vi "ppanel_DO_get_current_count_rates.vi"(8 "error in (no error)":errorcluster, 11 "hydraharp_panel in":refnum<class "picoharp_panel.lvclass">) -> (0 "error out":errorcluster, 3 "hydraharp_panel out":refnum<class "picoharp_panel.lvclass">)   [LabVIEW 2015, in "picoharp_panel.lvclass"]
uses:
  picoharp_panel.lvclass
  picoharp/picoharp.lvclass
  UI/panel_class/panel.lvclass
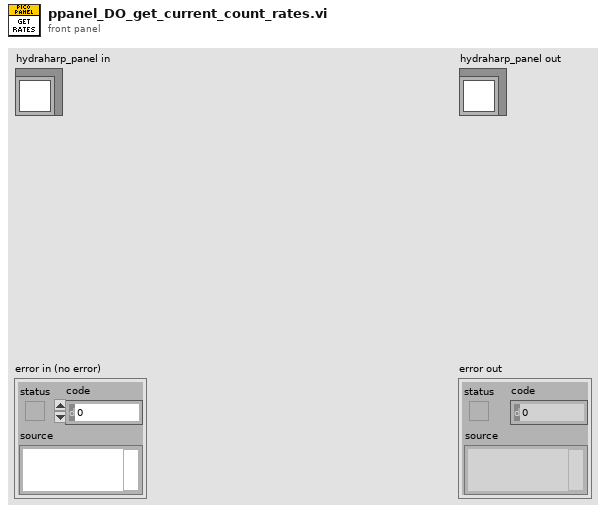
[diagram p1: front panel]
types:
  T1 = typedef "hydraharp_count_rates.ctl" = cluster{"channel_rates":i32[], "sync_rate":i32}
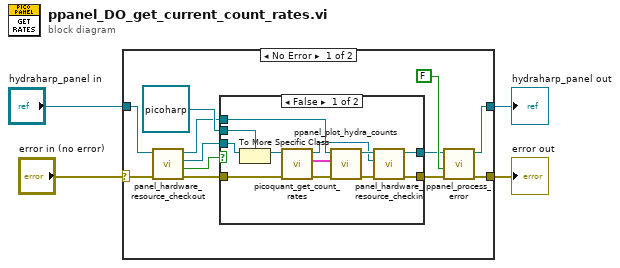
[diagram p0: block diagram]
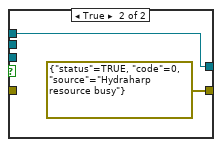
[diagram p2: hidden frame]
diagram:
  n1 = case shown="No Error" "error in (no error)" {
    selector: "error in (no error)" -> [w15 w32]
    tunnel: [w5 w32] -> w3
    tunnel: [w6 w31] -> w1
    tunnel: "hydraharp_panel in" -> [w16 w31]
    frame No Error {
      n2 = call "panel_hardware_resource_checkout.vi"("error in (no error)"=w15, "panel in"=w16) -> ("error out"=w10:errorcluster, "timed out?"=w14:bool, "hardware.lvclass"=w13:refnum<class "hardware.lvclass">, "panel out"=w11:refnum<class "picoharp_panel.lvclass">)  [unwired: 6 in]
      n3 = case shown="False" w14 {
        tunnel: w13 -> [w28 _]
        tunnel: refnum<class "picoharp.lvclass"> refnum ("picoharp.lvclass") -> [w27 _]
        tunnel: w11 -> [w26 w29]
        tunnel: w10 -> [w21 _]
        tunnel: [w22 errorcluster {"status"=TRUE, "code"=0, "source"="Hydraharp resource busy"} ("error out")] -> w8
        tunnel: [w23 w29] -> w7
        frame False {
          n4 = To More Specific Class(target class=w27, reference=w28) -> (specific class reference=w18:refnum<class "picoharp.lvclass">)  [unwired: 1 in, 1 out]
          n5 = call-dynamic "picoquant_get_count_rates.vi"("error in (no error)"=w21, "picoharp in"=w18) -> ("error out"=w20:errorcluster, "count_rates"=w19:T1, "picoharp out"=w17:refnum<class "picoharp.lvclass">)  [unwired: 7 in]
          n6 = call "ppanel_plot_hydra_counts.vi"("error in (no error)"=w20, "count_rates"=w19, "hydraharp_panel in"=w26) -> ("error out"=w25:errorcluster, "hydraharp_panel out"=w24:refnum<class "picoharp_panel.lvclass">)  [unwired: 7 in]
          n7 = call "panel_hardware_resource_checkin.vi"("error in (no error)"=w25, "hardware.lvclass"=w17, "panel in"=w24) -> ("error out"=w22:errorcluster, "panel out"=w23:refnum<class "picoharp_panel.lvclass">)  [unwired: 7 in]
        }
        frame True {
        }
      }
      n8 = call "ppanel_process_error.vi"("error in (no error)"=w8, "update_status"=FALSE, "hydraharp_panel in"=w7) -> ("error out"=w5:errorcluster, "hydraharp_panel out"=w6:refnum<class "picoharp_panel.lvclass">)  [unwired: 7 in]
    }
    frame Error {
    }
  }
  "error out" <- w3
  "hydraharp_panel out" <- w1
